vi "Get StartPoint.vi"(8 "error in (no error)":errorcluster, 11 "Line Border in":refnum<class "Line Border.lvclass">) -> (0 "error out":errorcluster, 2 "StartPoint":cluster{"x":i16, "y":i16}, 3 "Line Border out":refnum<class "Line Border.lvclass">)   [LabVIEW 2015, in "Line Border.lvclass"]
uses:
  Line Border.lvclass
  Line Border.lvclass/Line Border.ctl
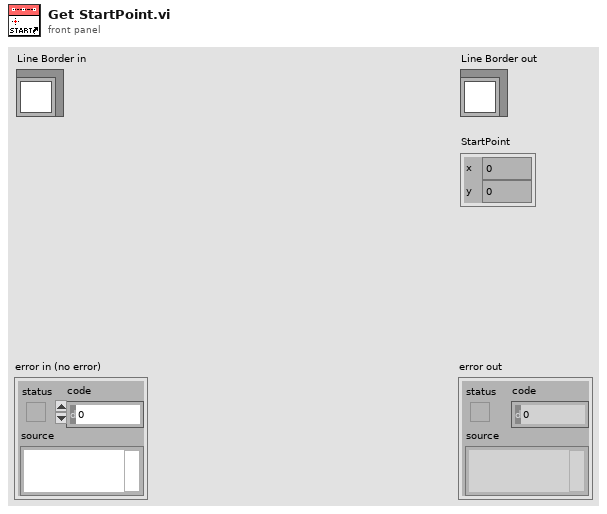
[diagram p1: front panel]
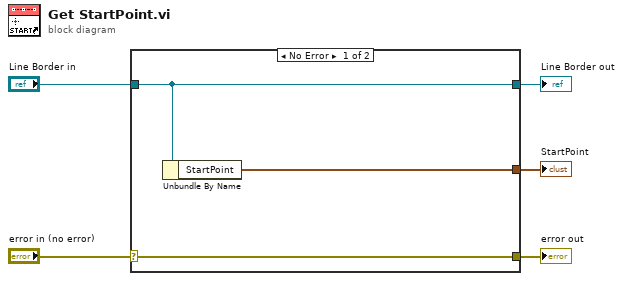
[diagram p0: block diagram]
diagram:
  n1 = case shown="No Error" "error in (no error)" {
    selector: "error in (no error)" -> [w8 w9]
    tunnel: [w8 w9] -> w4
    tunnel: [w7 w10] -> w2
    tunnel: "Line Border in" -> [w7 w10]
    tunnel: [w6 _] -> w1
    frame No Error {
      n2 = Unbundle By Name(w7) -> ("StartPoint"=w6:cluster{"x":i16, "y":i16})
    }
    frame Error {
    }
  }
  "error out" <- w4
  "Line Border out" <- w2
  "StartPoint" <- w1
